vi "Configure Modulation Pulse Time.vi"(8 "error in (no error)":errorcluster, 10 "pulse time, s":dbl=1.0, 11 "HFP Gen in":refnum<class "PL HFP Generator.lvclass">) -> (0 "error out":errorcluster, 3 "HFP Gen out":refnum<class "PL HFP Generator.lvclass">)   [LabVIEW 2015, in "PL HFP Generator.lvclass"]
doc: "Configures modulation pulse time (for Plasma GK series)"
uses:
  PL HFP Generator.lvclass
  PL HFP Generator.lvclass/PL HFP Generator.ctl
  <vilib>/plasmapper/PL Modbus Client/PL Modbus Client.lvclass
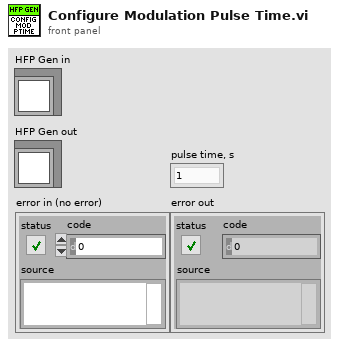
[diagram p1: front panel]
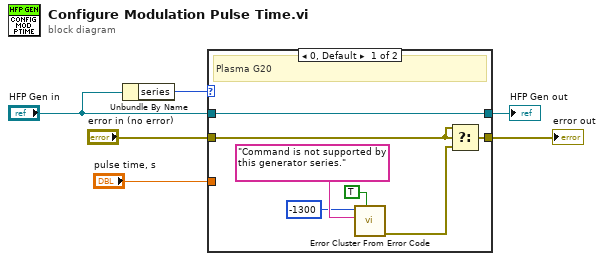
[diagram p0: block diagram]
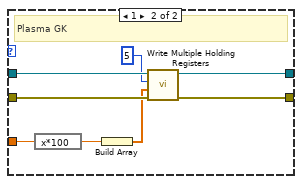
[diagram p2: hidden frame]
diagram:
  n1 = Unbundle By Name("HFP Gen in") -> ("series"=w2:u16)
  n2 = case shown="0, Default" w2 {
    tunnel: [w13 w21] -> w6
    tunnel: [w11 w20] -> w5
    tunnel: "error in (no error)" -> [w12 w19]
    tunnel: "HFP Gen in" -> [w13 w18]
    tunnel: "pulse time, s" -> [_ w14]
    frame 0, Default {
      # "Plasma G20"
      n3 = call <vilib>:"Error Cluster From Error Code.vi"("show call chain? (False)"=TRUE, "error message (\"\")"="Command is not supported by this generator series." ("format string"), "error code (0)"=-1300) -> ("error out"=w7:errorcluster)  [unwired: 6 in]
      n4 = Select(t=w12, s=w12, f=w7) -> (s? t:f=w11:errorcluster)
    }
    frame 1 {
      # "Plasma GK"
      n5 = expression code="x*100"(w14) -> (w15:dbl)
      n6 = Build Array(w15) -> (w16:dbl[])
      n7 = call <vilib>:"Write Multiple Holding Registers.vi"("error in (no error)"=w19, "values"=w16, "address"=u16 5, "MODBUS in"=w18) -> ("error out"=w20:errorcluster, "MODBUS out"=w21:refnum<class "PL HFP Generator.lvclass">)  [unwired: 6 in]
    }
  }
  "HFP Gen out" <- w6
  "error out" <- w5
